vi "Scan For Closed Key.vi"(8 "error in (no error)":errorcluster, 11 "VISA Refnum in":refnum<visa-resource-name>) -> (0 "error out":errorcluster, 1 "unsigned byte array":u8[](array[numeric]), 2 "Pass":bool, 3 "VISA Refnum out":refnum<visa-resource-name>)   [LabVIEW 2013]
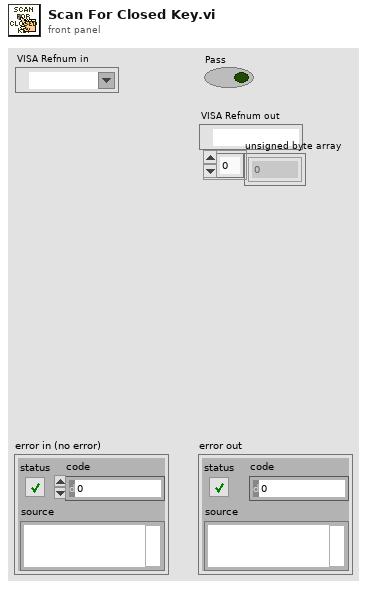
[diagram p1: front panel]
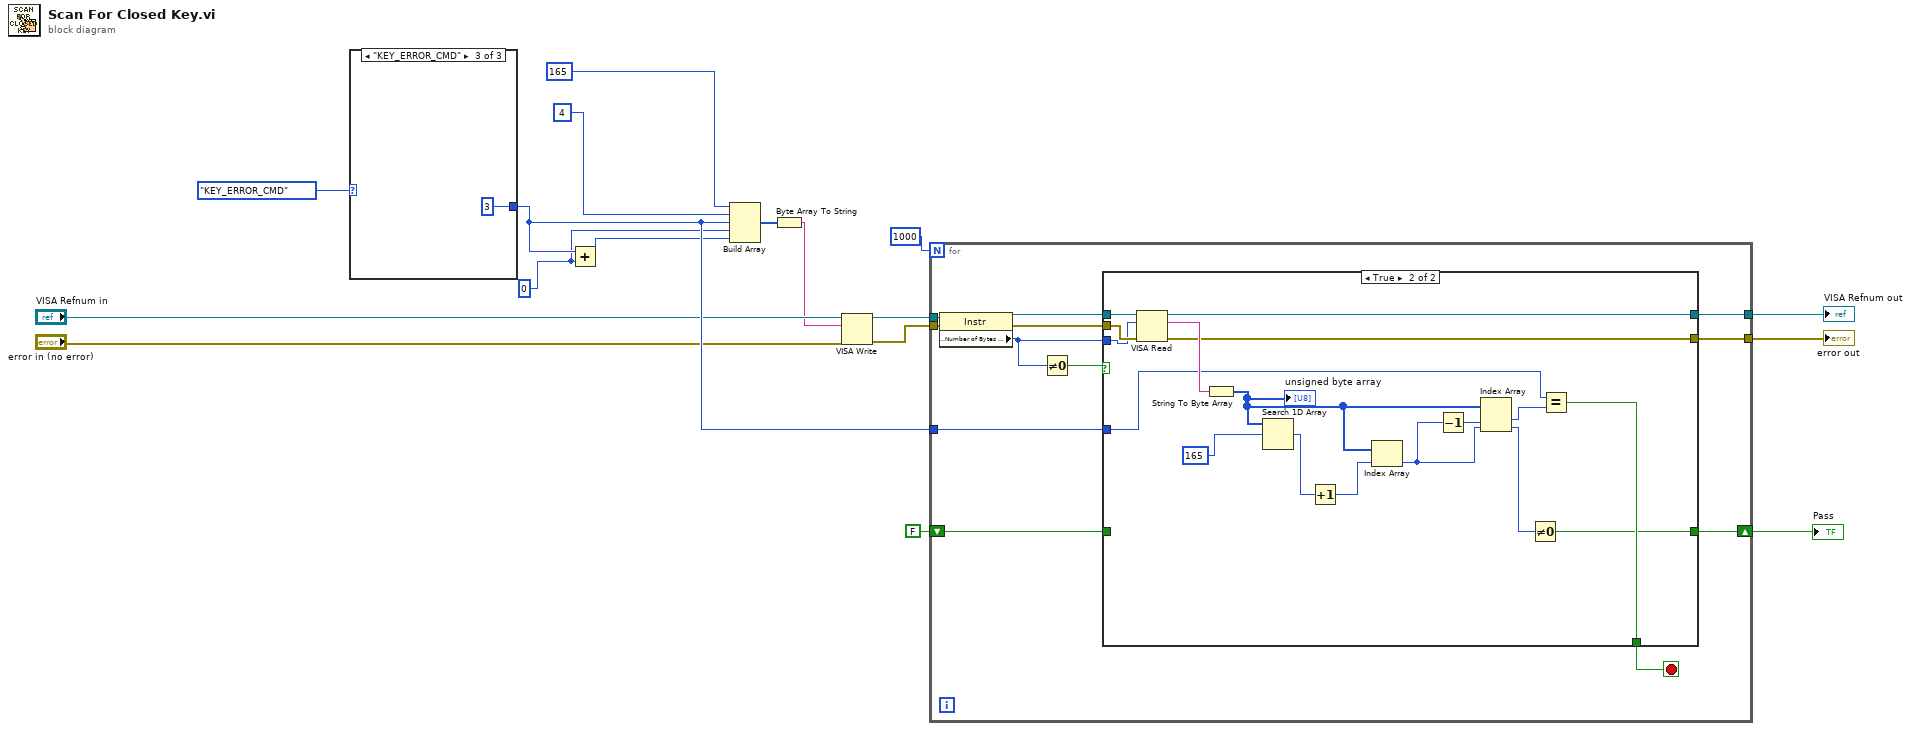
[diagram p0: block diagram]
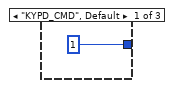
[diagram p3: hidden frame]
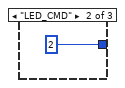
[diagram p4: hidden frame]
diagram:
  w2 = 0
  n1 = case shown="\"KEY_ERROR_CMD\"" enum16{"KYPD_CMD", "LED_CMD", "KEY_ERROR_CMD"}."KEY_ERROR_CMD" ("CMD") {
    tunnel: [1 2 3] -> w16
    frame "KYPD_CMD", Default {
    }
    frame "LED_CMD" {
    }
    frame "KEY_ERROR_CMD" {
    }
  }
  n2 = Add(x=w16, y=w2) -> (x+y=w4:i32)
  n3 = Build Array(u8 165, u8 4, w16, w2, w4) -> (w7:i32[])
  n4 = Byte Array To String(unsigned byte array=w7) -> (string=w3:string)
  n5 = VISA Write(VISA resource name="VISA Refnum in", write buffer=w3, error in (no error)="error in (no error)") -> (VISA resource name out=w11:refnum<visa-resource-name>, error out=w12:errorcluster)  [unwired: 1 out]
  n6 = for {
    N: 1000 -> [_]
    tunnel: w11 -> [w32]
    tunnel: w12 -> [w31]
    tunnel: [w26] -> w14
    tunnel: [w25] -> w13
    tunnel: w16 -> [w23]
    shift-right: [w22] -> w17
    shift-left: FALSE -> [w21]
    stop <- w24 stop-if-true
    n7 = property class="Instr"(reference=w32, error in=w31) -> (reference out=w29:refnum<visa-resource-name>, error out=w28:errorcluster, "Serial Settings:Number of Bytes at Serial Port"=w27:u32)
    n8 = Not Equal To 0?(x=w27) -> (x != 0?=w30:bool)
    n9 = case shown="True" w30 {
      tunnel: w29 -> [w34 w51]
      tunnel: w28 -> [_ w50]
      tunnel: w27 -> [_ w49]
      tunnel: [w34 w47] -> w26
      tunnel: [_ w46] -> w25
      tunnel: [_ w37] -> w24
      tunnel: w23 -> [_ w38]
      tunnel: [w33 w35] -> w22
      tunnel: w21 -> [w33 _]
      frame False {
      }
      frame True {
        n10 = VISA Read(VISA resource name=w51, byte count=w49, error in (no error)=w50) -> (VISA resource name out=w47:refnum<visa-resource-name>, read buffer=w48:string, error out=w46:errorcluster)  [unwired: 1 out]
        n11 = String To Byte Array(string=w48) -> (unsigned byte array=w42:u8[])
        "unsigned byte array" <- w42
        n12 = Search 1D Array(1D array=w42, element=u8 165) -> (index of element=w44:i32)  [unwired: 1 in]
        n13 = Increment(x=w44) -> (x+1=w43:i32)
        n14 = Index Array(array=w42, index=w43) -> (element=w40:u8)
        n15 = Decrement(x=w40) -> (x-1=w41:u8)
        n16 = Index Array(array=w42, index #1=w41, index #2=w40) -> (element #1=w39:u8, element #2=w36:u8)
        n17 = Not Equal To 0?(x=w36) -> (x != 0?=w35:bool)
        n18 = Equal?(x=w38, y=w39) -> (x = y?=w37:bool)
      }
    }
  }
  "Pass" <- w17
  "VISA Refnum out" <- w14
  "error out" <- w13
